vi "ZEROMQ_S4GUI.vi"() -> ()   [LabVIEW 2018]
uses:
  RxTx/RxTx.lvclass
  <vilib>/addons/zeromq/socket_type.ctl
  <vilib>/addons/zeromq/socket_options.ctl
  <vilib>/addons/zeromq/zmq_socket.lvclass
  <vilib>/addons/zeromq/zmq_context.lvclass
  <vilib>/addons/zeromq/zeromq.lvlib
panel:
  in  "Stop Button":bool
  in  "RxTx.lvclass":refnum<class "RxTx.lvclass">
  out "error out":errorcluster
  out "error out 3":errorcluster
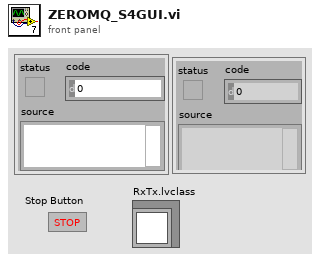
[diagram p1: front panel]
types:
  T1 = typedef "zeromq.lvlib/socket_options.ctl" = enum8{"NONE", "ZMQ_HWM", "<2>", "ZMQ_SWAP", "ZMQ_AFFINITY", "ZMQ_ROUTING_ID", "ZMQ_SUBSCRIBE", "ZMQ_UNSUBSCRIBE", "ZMQ_RATE", "ZMQ_RECOVERY_IVL", "ZMQ_MCAST_LOOP", "ZMQ_SNDBUF", "ZMQ_RCVBUF", "ZMQ_RCVMORE", "ZMQ_FD", "ZMQ_EVENTS", "ZMQ_TYPE", "ZMQ_LINGER", "ZMQ_RECONNECT_IVL", "ZMQ_BACKLOG", "ZMQ_RECOVERY_IVL_MSEC", "ZMQ_RECONNECT_IVL_MAX", "ZMQ_MAXMSGSIZE", "ZMQ_SNDHWM", "ZMQ_RCVHWM", "ZMQ_MULTICAST_HOPS", "<26>", "ZMQ_RCVTIMEO", "ZMQ_SNDTIMEO", "<29>", "<30>", "ZMQ_IPV4ONLY", "ZMQ_LAST_ENDPOINT", "ZMQ_ROUTER_MANDATORY", "ZMQ_TCP_KEEPALIVE", "ZMQ_TCP_KEEPALIVE_CNT", "ZMQ_TCP_KEEPALIVE_IDLE", "ZMQ_TCP_KEEPALIVE_INTVL", "ZMQ_TCP_ACCEPT_FILTER", "ZMQ_IMMEDIATE", "ZMQ_XPUB_VERBOSE", "ZMQ_ROUTER_RAW", "ZMQ_IPV6", "ZMQ_MECHANISM", "ZMQ_PLAIN_SERVER", "ZMQ_PLAIN_USERNAME", "ZMQ_PLAIN_PASSWORD", "ZMQ_CURVE_SERVER", "ZMQ_CURVE_PUBLICKEY", "ZMQ_CURVE_SECRETKEY", "ZMQ_CURVE_SERVERKEY", "ZMQ_PROBE_ROUTER", "ZMQ_REQ_CORRELATE", "ZMQ_REQ_RELAXED", "ZMQ_CONFLATE", "ZMQ_ZAP_DOMAIN", "ZMQ_ROUTER_HANDOVER", "ZMQ_TOS", "ZMQ_IPC_FILTER_PID", "ZMQ_IPC_FILTER_UID", "ZMQ_IPC_FILTER_GID", "ZMQ_CONNECT_ROUTING_ID", "ZMQ_GSSAPI_SERVER", "ZMQ_GSSAPI_PRINCIPAL", "ZMQ_GSSAPI_SERVICE_PRINCIPAL", "ZMQ_GSSAPI_PLAINTEXT", "ZMQ_HANDSHAKE_IVL", "<67>", "ZMQ_SOCKS_PROXY", "ZMQ_XPUB_NODROP", "ZMQ_BLOCKY", "ZMQ_XPUB_MANUAL", "ZMQ_XPUB_WELCOME_MSG", "ZMQ_STREAM_NOTIFY", "ZMQ_INVERT_MATCHING", "ZMQ_HEARTBEAT_IVL", "ZMQ_HEARTBEAT_TTL", "ZMQ_HEARTBEAT_TIMEOUT", "ZMQ_XPUB_VERBOSER", "ZMQ_CONNECT_TIMEOUT", "ZMQ_TCP_MAXRT", "ZMQ_THREAD_SAFE", "<82>", "<83>", "ZMQ_MULTICAST_MAXTPDU", "ZMQ_VMCI_BUFFER_SIZE", "ZMQ_VMCI_BUFFER_MIN_SIZE", "ZMQ_VMCI_BUFFER_MAX_SIZE", "ZMQ_VMCI_CONNECT_TIMEOUT", "ZMQ_USE_FD", "ZMQ_GSSAPI_PRINCIPAL_NAMETYPE", "ZMQ_GSSAPI_SERVICE_PRINCIPAL_NAMETYPE", "ZMQ_BINDTODEVICE", "ZMQ_ZAP_ENFORCE_DOMAIN", "ZMQ_LOOPBACK_FASTPATH", "ZMQ_METADATA", "ZMQ_MULTICAST_LOOP", "ZMQ_ROUTER_NOTIFY"}
  T2 = typedef "zeromq.lvlib/socket_type.ctl" = enum8{"ZMQ_PAIR", "ZMQ_PUB", "ZMQ_SUB", "ZMQ_REQ", "ZMQ_REP", "ZMQ_DEALER", "ZMQ_ROUTER", "ZMQ_PULL", "ZMQ_PUSH", "ZMQ_XPUB", "ZMQ_XSUB", "ZMQ_STREAM", "ZMQ_SERVER", "ZMQ_CLIENT", "ZMQ_RADIO", "ZMQ_DISH", "ZMQ_GATHER", "ZMQ_SCATTER", "ZMQ_DGRAM"}
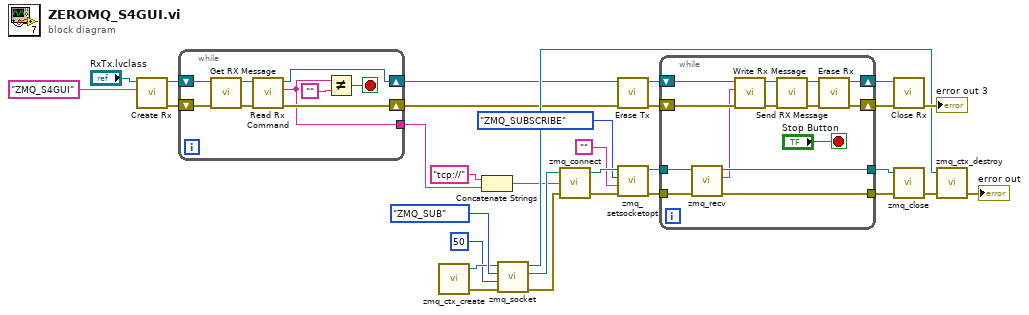
[diagram p0: block diagram]
diagram:
  n1 = call "Create Rx.vi"("Reader Name"="ZMQ_S4GUI" ("Writer Name"), "RxTx in"="RxTx.lvclass") -> ("error out"=w6:errorcluster, "RxTx out"=w7:refnum<class "RxTx.lvclass">)  [unwired: 8 in]
  n2 = while {
    shift-right: [w34] -> w9
    shift-left: w7 -> [w37]
    shift-right: [w33] -> w8
    shift-left: w6 -> [w38]
    tunnel: [w32] -> w2
    stop <- w39 stop-if-true
    n3 = call "Get RX Message.vi"("error in (no error)"=w38, "RxTx in"=w37) -> ("error out"=w36:errorcluster, "RxTx out"=w35:refnum<class "RxTx.lvclass">)  [unwired: 8 in]
    n4 = call "Read Rx Command.vi"("error in (no error)"=w36, "RxTx in"=w35) -> ("error out"=w33:errorcluster, "Rx Command"=w32:string, "RxTx out"=w34:refnum<class "RxTx.lvclass">)  [unwired: 7 in]
    n5 = Not Equal?(x=w32, y="") -> (x != y?=w39:bool)
  }
  n6 = call <vilib>:"zmq_ctx_create.vi"() -> ("error out"=w22:errorcluster, "context out"=w15:refnum<class "zmq_context.lvclass">)  [unwired: 4 in]
  n7 = Concatenate Strings("tcp://" ("endpoint"), w2) -> (w1:string)
  n8 = call <vilib>:"zmq_socket.vi"("error in"=w22, "linger (ms)"=50, "socket type"=socket_type."ZMQ_SUB", "context in"=w15) -> ("error out"=w21:errorcluster, "socket out"=w16:refnum<class "zmq_socket.lvclass">, "context out"=w11:refnum<class "zmq_context.lvclass">)  [unwired: 1 in]
  n9 = call <vilib>:"zmq_connect.vi"("error in"=w21, "endpoint"=w1, "socket in"=w16) -> ("error out"=w19:errorcluster, "socket out"=w20:refnum<class "zmq_socket.lvclass">)  [unwired: 1 in]
  n10 = call "Erase Tx.vi"("error in (no error)"=w8, "RxTx in"=w9) -> ("error out"=w5:errorcluster, "RxTx out"=w4:refnum<class "RxTx.lvclass">)  [unwired: 8 in]
  n11 = call <vilib>:"zmq_setsocketopt.vi"("error in"=w19, "value"="", "option"=socket_options."ZMQ_SUBSCRIBE", "socket in"=w20) -> ("error out"=w13:errorcluster, "socket out"=w12:refnum<class "zmq_socket.lvclass">)  [unwired: 2 in]
  n12 = while {
    shift-right: [w50] -> w26
    shift-left: w4 -> [w44]
    shift-right: [w49] -> w25
    shift-left: w5 -> [w45]
    tunnel: w12 -> [w54]
    tunnel: w13 -> [w53]
    tunnel: [w52] -> w30
    tunnel: [w42] -> w29
    stop <- "Stop Button" stop-if-true
    n13 = call <vilib>:"zmq_recv.vi"("error in"=w53, "socket in"=w54) -> ("error out"=w42:errorcluster, "data"=w43:string, "socket out"=w52:refnum<class "zmq_socket.lvclass">)  [unwired: 3 in, 2 out]
    n14 = call "Write Rx Message.vi"("error in (no error)"=w45, "Rx Message"=w43, "RxTx in"=w44) -> ("error out"=w46:errorcluster, "RxTx out"=w47:refnum<class "RxTx.lvclass">)  [unwired: 7 in]
    n15 = call "Send RX Message.vi"("error in (no error)"=w46, "RxTx in"=w47) -> ("error out"=w48:errorcluster, "RxTx out"=w51:refnum<class "RxTx.lvclass">)  [unwired: 8 in]
    n16 = call "Erase Rx.vi"("error in (no error)"=w48, "RxTx in"=w51) -> ("error out"=w49:errorcluster, "RxTx out"=w50:refnum<class "RxTx.lvclass">)  [unwired: 8 in]
  }
  n17 = call "Close Rx.vi"("error in (no error)"=w25, "RxTx in"=w26) -> ("error out"=→"error out 3":errorcluster)  [unwired: 8 in, 1 out]
  n18 = call <vilib>:"zmq_close.vi"("error in"=w29, "socket"=w30) -> ("error out"=w31:errorcluster)  [unwired: 3 in]
  n19 = call <vilib>:"zmq_ctx_destroy.vi"("error in"=w31, "context in"=w11) -> ("error out"=→"error out":errorcluster)  [unwired: 3 in]
